vi "SandE main loop.vi"(1 "Loop ID":T1, 11 "error in (no error)":errorcluster) -> ()   [LabVIEW 2011]
doc: "This VI contains an engine that logs errors and events to file."
uses:
  Application Structure/Loop ID.ctl
  emi cndiates/E&S/Monitor/Actino S&E monitor.ctl
  emi Lib/System 01/0 - General/App/Loop control 2/Private/_emi_ SMLoop start condition.vi
  emi Lib/System 01/0 - General/App/Loop control 2/Private/_emi_ SMLoop Error Check.vi
  emi Lib/Basic/0 - General/Error/emi_Is Error.vi
  emi Lib/System 01/0 - General/App/Loop control 2/Private/_emi_SMLoop Register new.vi
  emi Lib/System 01/0 - General/S&E reporting/emi_Send S&E Error message.vi
  emi Lib/Basic/0 - General/Error/emi_ Is Error state.vi
  emi Lib/System 01/0 - General/emi_Read System ID.vi
  emi Lib/System 01/0 - General/App/Loop control/Private/_emi_GFV Loop Linking.vi
  emi Lib/System 01/0 - General/App/Loop control/Private/_emi_GFV Loop Enable.vi
  emi Lib/System 01/0 - General/App/Loop control 2/Private/_emi_ SMLoop Restart.vi
  emi Lib/System 01/0 - General/App/Private/_emi_GFV App Close.vi
  emi Lib/System 01/0 - General/App/Loop control 2/Private/_emi_ SMLoop Restart Counter.vi
  emi Lib/System 01/0 - General/App/Loop control/Private/_emi_GFV Loop Running.vi
  emi Lib/System 01/0 - General/Private/_emi_GFV System ID.vi
  emi Lib/System 01/0 - General/S&E reporting/Private/_emi_S&E Q Generator.vi
  <vilib>/Utility/error.llb/Clear Errors.vi
  emi Lib/System 01/0 - General/App/Loop control/Private/_emi_GFV stop a loop so it can reset.vi
  emi Lib/Basic/0 - General/App/Version/Private/_emi_Version Holder.vi
  emi Lib/Basic/0 - General/Time/Private/emi_Time offset holder.vi
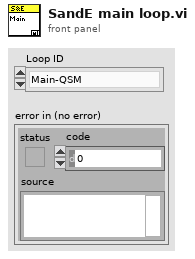
[diagram p1: front panel]
types:
  T1 = typedef "Loop ID.ctl" = enum16{"Main-QSM", "Main-Dialog", "Main-Ind Upd", "Main-Graph Upd", "Main-Debug", "Main-DebugW1", "Main-DebugW2", "Main-SE Handler", "Interface-PCP", "Interface-CANbus", "Interface-Modem", "Var Handling-Beat", "Var Handling-From PCP", "Var Handling-File storage", "Var Handling-From Simulator", "GUI-GrphW Mast", "GUI-GrphW Slav", "SIM-Tool W1", "SIM-Tool W2", "Alm-Sound", "LEIN-motor", "Tool data gatherer Qer", "Tool Data LEIN STAT2 dekoder", "Indicator Value Update", "Tool STAT2 dedicated reader", "Tool ID handler", "Detail View L1", "Detail View L2", "Main display enable view", "Sequence runner", "Voltage setpoint", "Resistance setpoint", "Stroker Wizard L1", "Stroker Wizard L2", "Alarm Handling", "Annotations Tip Strip", "Magna Interface", "Modem Status", "Var Handling - Modem Status", "Power interface detector"}
  T2 = typedef "Actino S&E monitor.ctl" = enum16{"GET(type history)", "SET S&E", "(Re)Init", "Get Error state", "Get  Alarm state", "Get All", "Get last  250", "Get Alarm History"}
  T3 = typedef "_emi_ SMLoop sates.ctl" = enum16{"Init", "Standby", "Start", "Normal Operation", "Stop", "Error Handling", "End", "Post"}
  T4 = typedef "Project infor with project path.ctl" = cluster{"Project path":path, "data":T5, "Comment":string}
  T5 = typedef "Project in icluster.ctl" = cluster{"Job and Site":T6, "Tool":T8, "Run Information":T9}
  T6 = typedef "Job and site cluster.ctl" = cluster{"Project Number":string, "Client Company":string, "Country":T7, "Field":string, "Rig":string, "Well":string}
  T7 = typedef "List of all contrys(combo box).ctl" = string
  T8 = typedef "Tool registration ID.ctl" = cluster{"Tractor type":string, "Tool":string, "Serial #":string}
  T9 = typedef "Run Information.ctl" = cluster{"Active Run":bool, "String Check Rec":bool, "Run Number":i32, "Time of File Start":string}
  T10 = typedef "emi_Version Info.ctl" = cluster{"Name":string, "Major":i16, "Minor":i16, "Fix":i16, "Build":i32, "Type":enum16{"Alfa", "Beta", "Stable"}, "Dev":bool, "Version Name":string, "Date":timestamp}
  T11 = typedef "_emi_ S&E Message.ctl" = cluster{"Type":T12, "Originate time":dbl, "System":u8, "Loop":u16, "Sub ID":u16, "Elevated priority":bool, "E&S Message content":variant}
  T12 = typedef "_emi_ S&E Message type.ctl" = enum16{"Error/Warning", "Note", "Debug", "Event", "Alarm Analog", "Alarm Digital", "Annotation"}
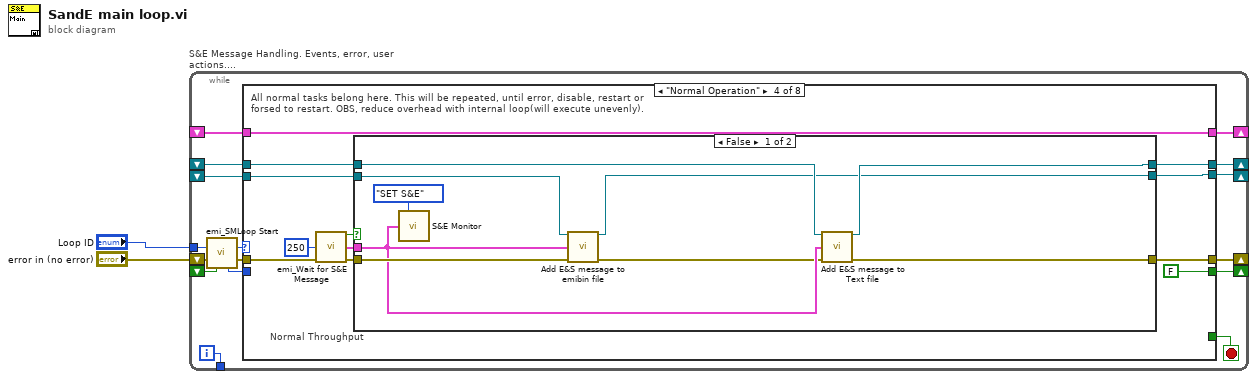
[diagram p0: block diagram]
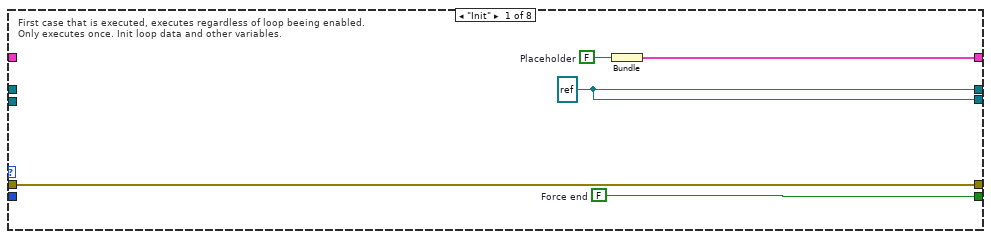
[diagram p2: hidden frame]
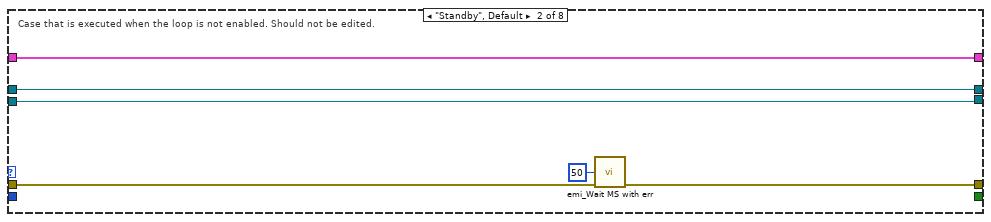
[diagram p3: hidden frame]
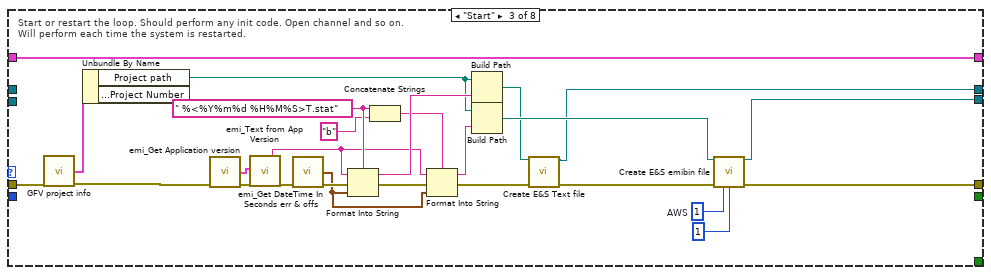
[diagram p4: hidden frame]
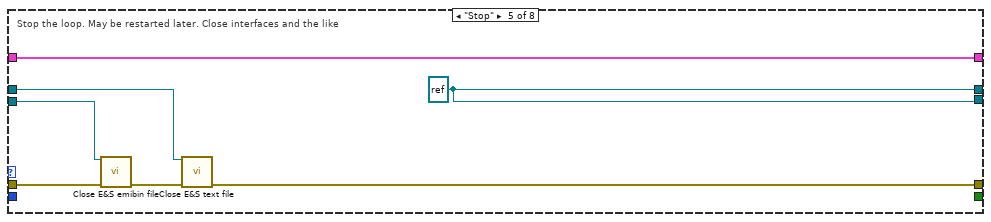
[diagram p6: hidden frame]
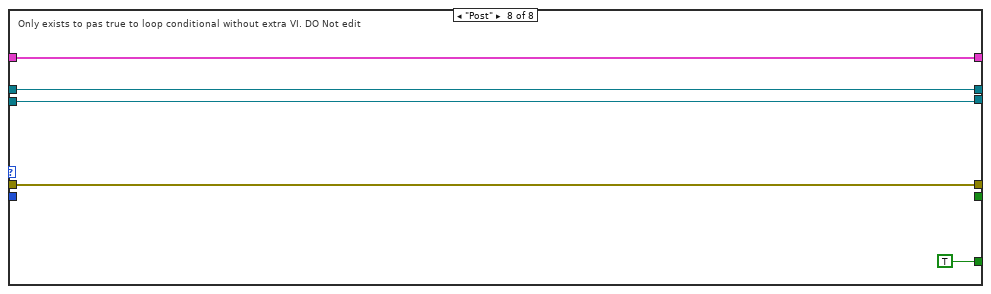
[diagram p9: hidden frame]
diagram:
  n1 = while "S&E Message Handling. Events, error, user actions...." {
    shift-right: [w18] -> _
    shift-left: _ -> [w14]
    shift-right: [w16] -> _
    shift-left: "error in (no error)" -> [w12]
    tunnel: [w15] -> _
    shift-right: [w13] -> _
    shift-left: _ -> [w8]
    tunnel: "Loop ID" -> [w9]
    shift-right: [w6] -> _
    shift-left: _ -> [w5]
    shift-right: [w4] -> _
    shift-left: _ -> [w3]
    i -> [w15]
    stop <- w17 stop-if-true
    n2 = call "emi_SMLoop Start.vi"("Loop ID"=w9, "error in (no error)"=w12, "Force Stop(F)"=w8) -> ("Loop command"=w10:T3, "error out"=w11:errorcluster, "Loop ID out"=w7:i32)  [unwired: 10 in]
    n3 = case shown="\"Normal Operation\"" w10 {
      tunnel: [w22 w26 w55 w65 w86 w90 w93 w98] -> w18
      tunnel: [_ _ _ _ _ _ _ TRUE] -> w17
      tunnel: w11 -> [w23 w28 w54 w67 w84 w89 w94 w99]
      tunnel: [w23 w27 w38 w66 w80 w89 w94 w99] -> w16
      tunnel: w14 -> [_ w26 w55 w65 w86 w90 w93 w98]
      tunnel: [w20 _ _ FALSE ("Force End") _ _ _ _] -> w13
      tunnel: w7 -> [_ _ _ _ _ _ _ _]
      tunnel: [w19 w25 w34 w62 w85 w88 w92 w96] -> w6
      tunnel: w5 -> [_ w25 _ w63 w82 w88 w92 w96]
      tunnel: [w19 w24 w39 w60 w85 w87 w91 w95] -> w4
      tunnel: w3 -> [_ w24 _ w61 w83 w87 w91 w95]
      frame "Init" {
        w19 = refnum<file> refnum ("refnum out")
        w20 = FALSE  # Force end
        w21 = FALSE  # Placeholder
        # "First case that is executed, executes regardless of loop beeing enabled.\nOnly executes once. Init loop data and other variables."
        n4 = Bundle("Placeholder"=w21) -> (w22:cluster{"Placeholder":bool})  [unwired: 1 in]
      }
      frame "Standby", Default {
        # "Case that is executed when the loop is not enabled. Should not be edited."
        n5 = call "emi_Wait MS with err.vi"("milliseconds to wait(0)"=u32 50, "error in (no error)"=w28) -> ("error out"=w27:errorcluster)  [unwired: 13 in]
      }
      frame "Start" {
        w31 = u16 1  # AWS
        w47 = " %<%Y%m%d %H%M%S>T.stat" ("format string")
        # "Start or restart the loop. Should perform any init code. Open channel and so on. \nWill perform each time the system is restarted."
        n6 = call "GFV project info.vi"("error in (no error)"=w54) -> ("Project info out"=w30:T4, "error out"=w49:errorcluster)  [unwired: 13 in]
        n7 = Unbundle By Name(w30) -> ("Project path"=w42:path)  [unwired: 1 out]
        n8 = call "emi_Get Application version.vi"("error in (no error)"=w49) -> ("Version Info out"=w53:T10, "error out"=w52:errorcluster)  [unwired: 12 in, 1 out]
        n9 = call "emi_Text from App Version.vi"("Version Info"=w53, "error in (no error)"=w52) -> ("Name"=w44:string, "error out"=w51:errorcluster)  [unwired: 8 in, 8 out]
        n10 = call "emi_Get DateTime In Seconds err & offs.vi"("error in (no error)"=w51) -> ("Time"=w36:timestamp, "error out"=w50:errorcluster)  [unwired: 13 in]
        n11 = Format Into String(format string=w47, initial string=w44, error in=w50, w36) -> (resulting string=w48:string, error out=w45:errorcluster)
        n12 = Concatenate Strings(w47, "b" ("string")) -> (w43:string)
        n13 = Format Into String(format string=w43, initial string=w44, error in=w45, w36) -> (resulting string=w41:string, error out=w37:errorcluster)
        n14 = Build Path(base path=w42, name or relative path=w48) -> (appended path=w33:path)
        n15 = Build Path(base path=w42, name or relative path=w41) -> (appended path=w40:path)
        n16 = call "Create E&S Text file.vi"("file path (use dialog)"=w33, "error in (no error)"=w37) -> ("refnum out"=w34:refnum<file>, "error out"=w35:errorcluster)  [unwired: 12 in]
        n17 = call "Create E&S emibin file.vi"("file path (use dialog)"=w40, "error in (no error)"=w35, "E&# File type ID(0, generic)"=w31, "E&S File type Version(0, Unset)"=u8 1) -> ("refnum out"=w39:refnum<file>, "error out"=w38:errorcluster)  [unwired: 10 in]
      }
      frame "Normal Operation" {
        # "Normal Throughput"
        # "All normal tasks belong here. This will be repeated, until error, disable, restart or\nforsed to restart. OBS, reduce overhead with internal loop(will execute unevenly)."
        n18 = call "emi_Wait for S&E Message.vi"("timeout in ms (5)"=250, "error in (no error)"=w67) -> ("timed out?"=w58:bool, "E&S Message"=w56:T11, "error out"=w57:errorcluster)  [unwired: 11 in]
        n19 = case shown="False" w58 {
          tunnel: [w75 w79] -> w66
          tunnel: w57 -> [w76 w79]
          tunnel: w56 -> [w72 _]
          tunnel: w63 -> [w74 w78]
          tunnel: [w73 w78] -> w62
          tunnel: w61 -> [w70 w77]
          tunnel: [w69 w77] -> w60
          frame False {
            n20 = call "S&E Monitor.vi"("Action(GET 250)"=Actino_S&E_monitor."SET S&E" ("Action(GET)"), "E&S Message in"=w72) -> ()  [unwired: 12 in, 2 out]
            n21 = call "Add E&S message to emibin file.vi"("refnum in"=w70, "E&S Message"=w72, "error in (no error)"=w76) -> ("refnum out"=w69:refnum<file>, "error out"=w68:errorcluster)  [unwired: 11 in]
            n22 = call "Add E&S message to Text file.vi"("refnum in"=w74, "E&S Message"=w72, "error in (no error)"=w68) -> ("refnum out"=w73:refnum<file>, "error out"=w75:errorcluster)  [unwired: 11 in]
          }
          frame True {
            # "Timeout"
          }
        }
      }
      frame "Stop" {
        w85 = refnum<file> refnum ("refnum out")
        # "Stop the loop. May be restarted later. Close interfaces and the like"
        n23 = call "Close E&S emibin file.vi"("refnum in"=w83, "error in (no error)"=w84) -> ("error out"=w81:errorcluster)  [unwired: 13 in]
        n24 = call "Close E&S text file.vi"("refnum in"=w82, "error in (no error)"=w81) -> ("error out"=w80:errorcluster)  [unwired: 13 in]
      }
      frame "Error Handling" {
        # "Loop automaticaly returns here after error is found. If error is cleared, Loop wil continue\nas normal(if was operative when error."
      }
      frame "End" {
        # "Only executes at application end has. Should performa any action the loop needs to finnish. \nExecutes only once."
      }
      frame "Post" {
        # "Only exists to pas true to loop conditional without extra VI. DO Not edit"
      }
    }
  }
